vi "Read Realsense Cam.vi"(8 "error in (no error)":errorcluster, 11 "Realsense Cam File Wrapper in":refnum<class "Realsense Cam File Wrapper.lvclass">) -> (0 "error out":errorcluster, 2 "Realsense Cam.lvclass":refnum<class "Realsense Cam.lvclass">, 3 "Realsense Cam File Wrapper out":refnum<class "Realsense Cam File Wrapper.lvclass">)   [LabVIEW 2018, in "Realsense Cam File Wrapper.lvclass"]
uses:
  Realsense Cam File Wrapper.lvclass
  Realsense Cam/Realsense Cam.lvclass
  Realsense Cam File Wrapper.lvclass/Realsense Cam File Wrapper.ctl
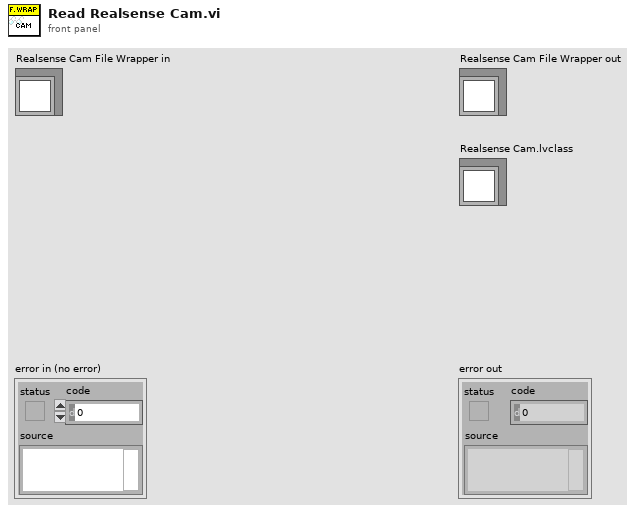
[diagram p1: front panel]
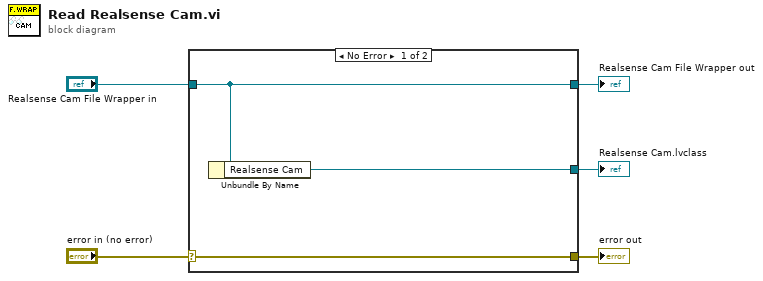
[diagram p0: block diagram]
diagram:
  n1 = case shown="No Error" "error in (no error)" {
    selector: "error in (no error)" -> [w8 w9]
    tunnel: [w8 w9] -> w4
    tunnel: [w7 w10] -> w2
    tunnel: "Realsense Cam File Wrapper in" -> [w7 w10]
    tunnel: [w6 _] -> w1
    frame No Error {
      n2 = Unbundle By Name(w7) -> ("Realsense Cam"=w6:refnum<class "Realsense Cam.lvclass">)
    }
    frame Error {
    }
  }
  "error out" <- w4
  "Realsense Cam File Wrapper out" <- w2
  "Realsense Cam.lvclass" <- w1
